vi "Viewer Status Message.vi"(8 "error in (no error)":errorcluster, 9 "Counts":dbl, 10 "Message":string, 11 "Application in":refnum<class "Application.lvclass">) -> (0 "error out":errorcluster, 3 "Application out":refnum<class "Application.lvclass">)   [LabVIEW 2023, in "Application.lvlib" / "Application.lvclass"]
uses:
  Application.lvclass
  Mode.ctl
  Application.lvclass/Application.ctl
  User Interface/Viewer Messages/Status Update Msg/Status Update Msg.lvclass/Status Update Msg.ctl
  <vilib>/ActorFramework/Message Enqueuer/Message Enqueuer.lvclass/Message Enqueuer.ctl
  <vilib>/ActorFramework/Message Enqueuer/Enqueue.vi
  User Interface/Viewer Messages/Status Update Msg/Status Update Msg.lvclass
  C:/Program Files/National Instruments/LabVIEW 2023/vi.lib/ActorFramework/Message/Message.lvclass
  Resources/GLOBAL/GLOBAL Time-critical.vi
  <vilib>/ActorFramework/Message Priority Queue/Priority Enqueue.vi
  Application.lvlib
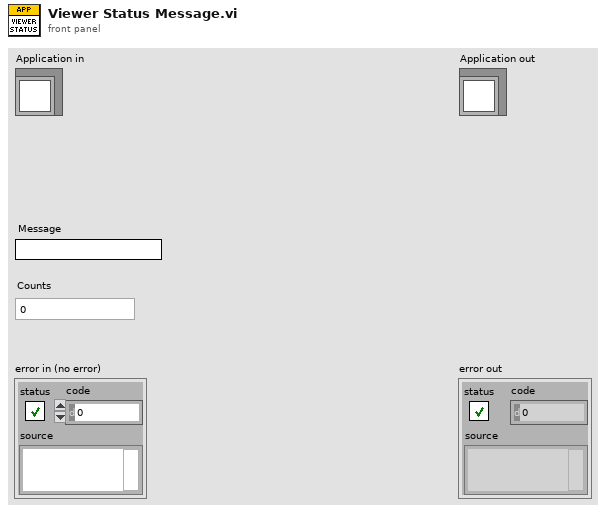
[diagram p1: front panel]
types:
  T1 = typedef "Application.lvlib/Mode.ctl" = enum16{"Idle", "Cancel", "Live", "Stream", "Autofocus", "Z-Stack", "Montage", "Saving", "Stage Scan", "Laser Adjust"}
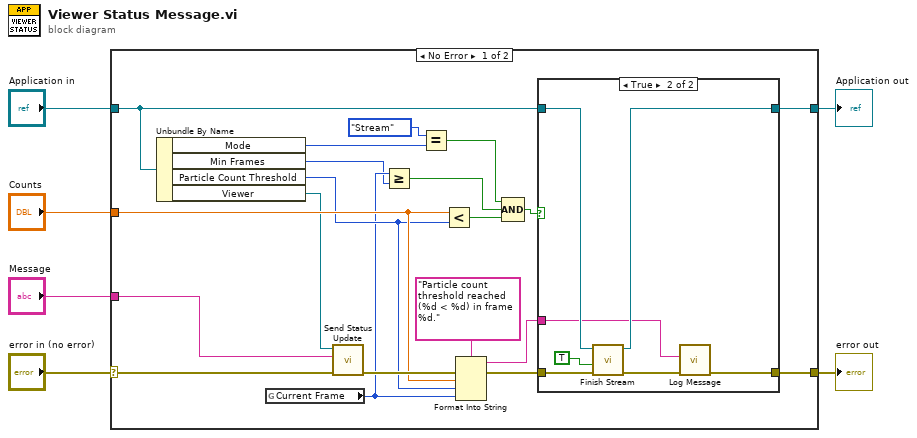
[diagram p0: block diagram]
diagram:
  n1 = case shown="No Error" "error in (no error)" {
    selector: "error in (no error)" -> [w26 w37]
    tunnel: [w24 w37] -> w5
    tunnel: [w22 w36] -> w3
    tunnel: "Application in" -> [w23 w36]
    tunnel: "Message" -> [w25 _]
    tunnel: "Counts" -> [w16 _]
    frame No Error {
      n2 = Unbundle By Name(w23) -> ("Mode"=w13:T1, "Min Frames"=w9:i32, "Particle Count Threshold"=w11:i32, "Viewer"=w14:refnum<class "Message Enqueuer.lvclass">)
      n3 = global read "GLOBAL Time-critical.vi" "Current Frame"() -> (w10:i32)
      n4 = call "Send Status Update.vi"("error in (no error)"=w26, "Message"=w25, "Message Enqueuer"=w14) -> ("error out"=w18:errorcluster)  [unwired: 7 in, 1 out]
      n5 = Greater Or Equal?(x=w10, y=w9) -> (x >= y?=w7:bool)
      n6 = Equal?(x=Mode."Stream" ("y"), y=w13) -> (x = y?=w8:bool)
      n7 = Less?(x=w16, y=w11) -> (x < y?=w20:bool)
      n8 = Format Into String(format string="Particle count threshold reached (%d < %d) in frame %d." ("input"), error in=w18, w16, w11, w10) -> (resulting string=w15:string, error out=w17:errorcluster)  [unwired: 1 in]
      n9 = Compound Arithmetic op=AND(w8, w7, w20) -> (w21:bool)
      n10 = case shown="True" w21 {
        tunnel: w17 -> [w27 w35]
        tunnel: [w27 w30] -> w24
        tunnel: w23 -> [w28 w34]
        tunnel: [w28 w33] -> w22
        tunnel: w15 -> [_ w29]
        frame False {
        }
        frame True {
          n11 = call-dynamic "Finish Stream.vi"("error in (no error)"=w35, "Save partial?"=TRUE, "Application in"=w34) -> ("error out"=w31:errorcluster, "Application out"=w33:refnum<class "Application.lvclass">)  [unwired: 7 in]
          n12 = call "Log Message.vi"("error constant"=w31, "input"=w29) -> ("error constant 2"=w30:errorcluster)  [unwired: 8 in, 1 out]
        }
      }
    }
    frame Error {
    }
  }
  "error out" <- w5
  "Application out" <- w3
